vi "calc_velocity.vi"(9 "Time per cell":i32, 10 "Path length":dbl, 11 "Neurons":u16) -> (3 "Velocity":dbl)   [LabVIEW 2011]
panel:
  in  "value":u16=1000
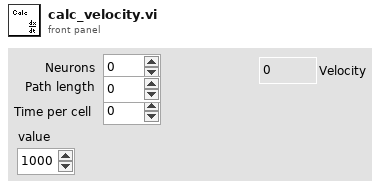
[diagram p1: front panel]
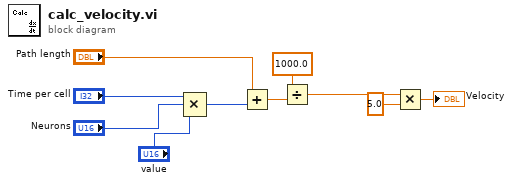
[diagram p0: block diagram]
diagram:
  n1 = Compound Arithmetic op=MULTIPLY("Time per cell", "Neurons", "value") -> (w6:i32)
  n2 = Add(x="Path length", y=w6) -> (x+y=w8:dbl)
  n3 = Divide(x=1000.0, y=w8) -> (x/y=w10:dbl)
  n4 = Multiply(x=w10, y=5.0) -> (x*y=→"Velocity":dbl)
